vi "AgilentAutoSignalCaptureBinary.vi"() -> ()   [LabVIEW 2016]
uses:
  AgilentControl.ctl
  Channel Config.ctl
  <vilib>/Waveform/WDTOps.llb/WDT Waveform Duration DBL.vi
  <instrlib>/Agilent 6000 Series/Agilent 6000 Series.lvlib
panel:
  out "File Errors":errorcluster
  in  "Shot Notes":string
  out "Last Shot Number":u32
  out "Num Events so far":i32
  out "Last Captured Waveform":waveform(dbl)[](graph)
  in  "Update Graph":bool
  out "Time per acq (ms)":dbl
  out "Elapsed Time (ms)":u32
  in  "Max Waves to capture":i32 min=0 max=1000000 step=1
  in  "Target Data Folder":path=path "C:/test"
  out "Close Error":errorcluster
  in  "stop":bool
  out "Agilent Control Out":T1={"Trig?"=FALSE, "VISA session"="", "Setup to Load"="CH1", "Timeout (ms)"=10000, "Desired Samp"=enum."100", "Captured Samp"=0, "Desired Channels"=[]}
  in  "Agilent Control In":T1={"Trig?"=FALSE, "VISA session"="Agilent6034A", "Setup to Load"="CH1", "Timeout (ms)"=10000, "Desired Samp"=enum."100", "Captured Samp"=2, "Desired Channels"=[]}
  out "Data Download Error":errorcluster[](array[cluster])
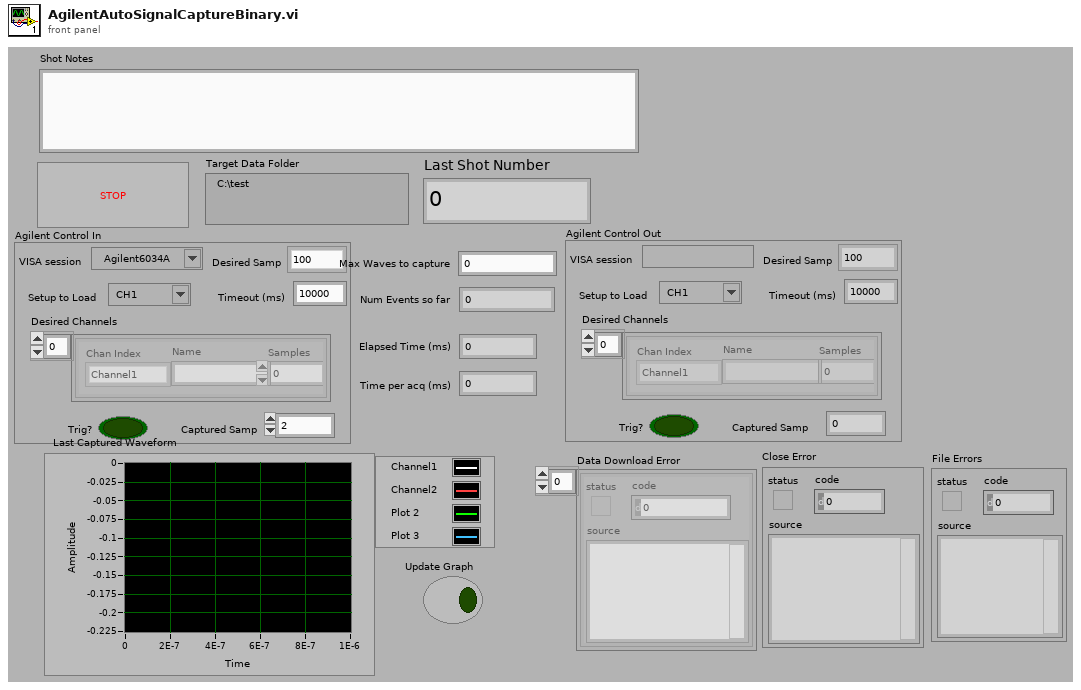
[diagram p1: front panel]
types:
  T1 = typedef "AgilentControl.ctl" = cluster{"Trig?":bool, "VISA session":refnum<visa-resource-name>, "Setup to Load":string, "Timeout (ms)":u32, "Desired Samp":enum32{"100", "250", "500", "1000", "2000", "5000", "10000", "20000", "50000", "100000", "200000", "500000", "1000000", "2000000", "4000000", "8000000"}, "Captured Samp":i32, "Desired Channels":T2[]}
  T2 = typedef "Channel Config.ctl" = cluster{"Chan Index":enum16{"Channel1", "Channel2", "Channel3", "Channel4", "MATH"}, "Name":string, "Samples":i32}
  T3 = enum16{"open", "replace", "create", "open or create", "replace or create", "replace or create with confirmation"}
  T4 = enum32{"100", "250", "500", "1000", "2000", "5000", "10000", "20000", "50000", "100000", "200000", "500000", "1000000", "2000000", "4000000", "8000000"}
  T5 = enum16{"Channel1", "Channel2", "Channel3", "Channel4", "MATH"}
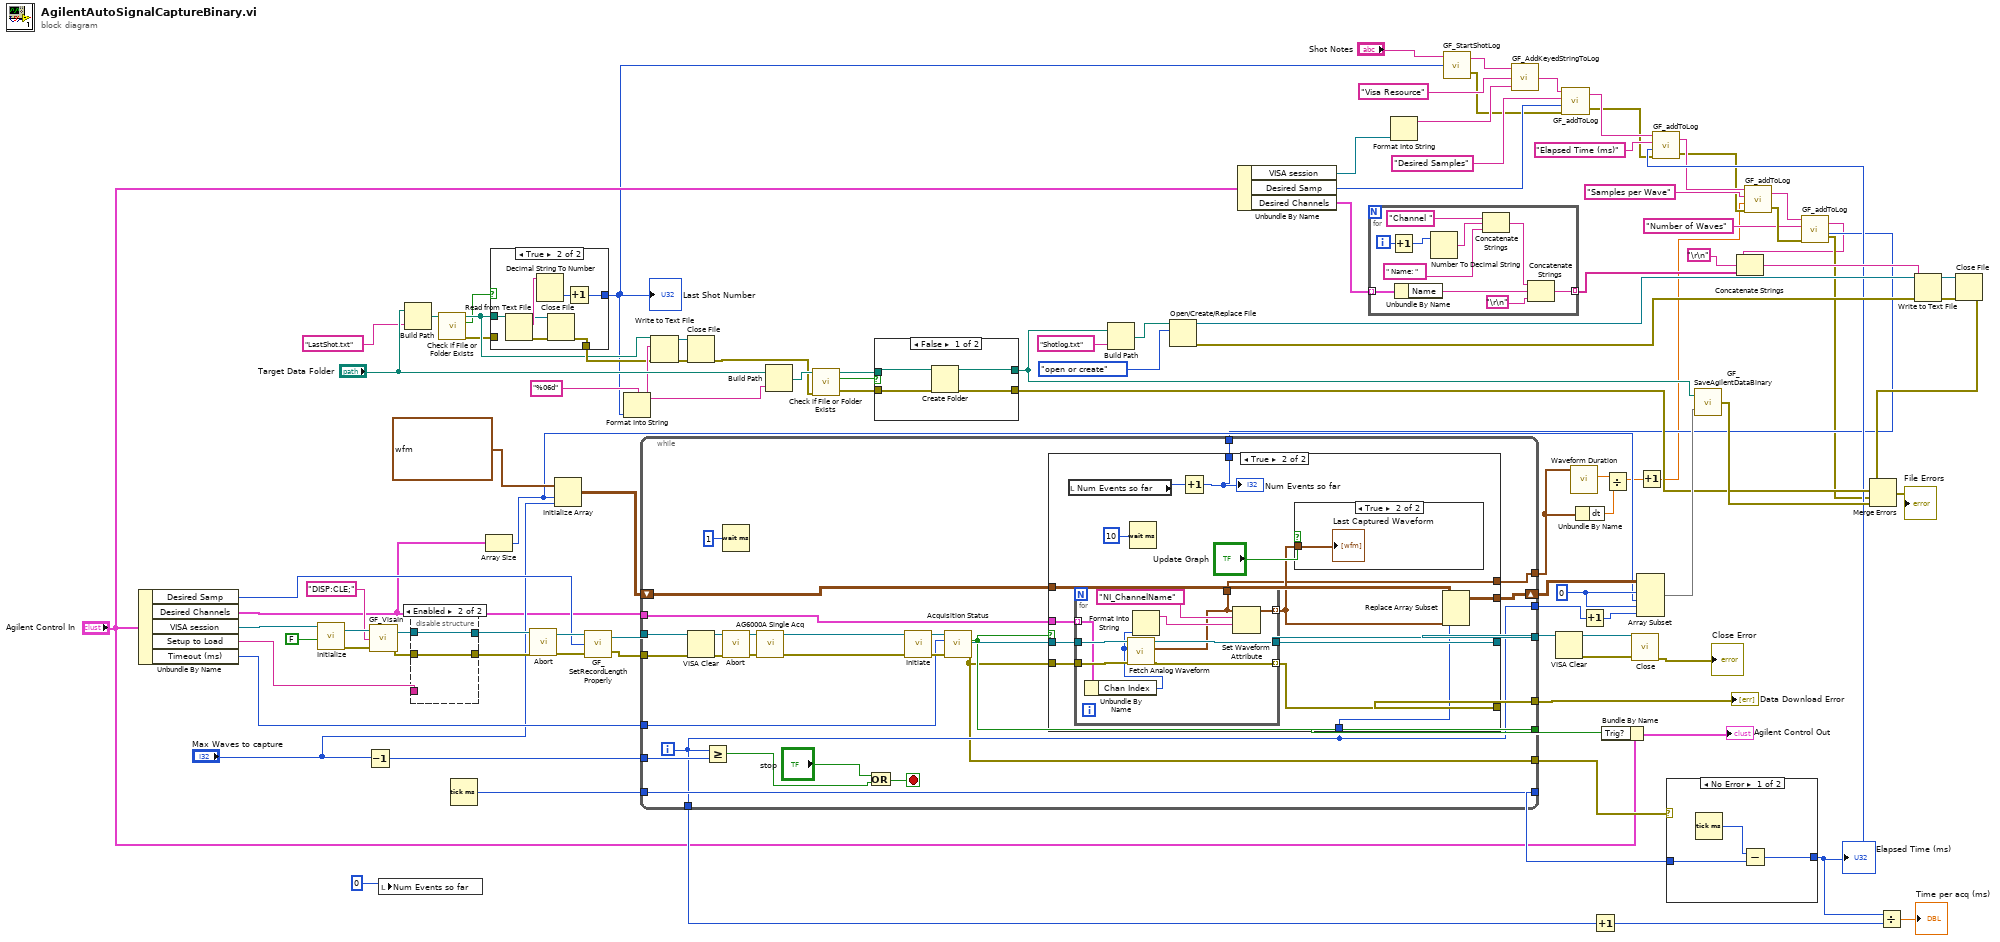
[diagram p0: block diagram]
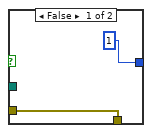
[diagram p2: hidden frame]
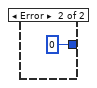
[diagram p4: hidden frame]
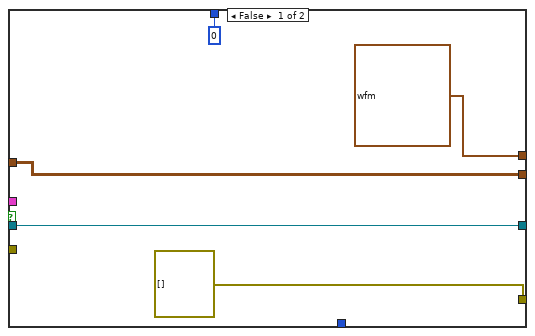
[diagram p5: hidden frame]
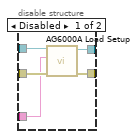
[diagram p7: hidden frame]
diagram:
  w64 = 0 ("index")
  n1 = Unbundle By Name("Agilent Control In") -> ("Desired Samp"=w75:T4, "Desired Channels"=w70:T2[], "VISA session"=w101:refnum<visa-resource-name>, "Setup to Load"=w99:string, "Timeout (ms)"=w98:u32)
  n2 = call <instrlib>:"Initialize.vi"("Reset? (T: Yes)"=FALSE, "VISA resource name"=w101) -> ("error out"=w90:errorcluster, "VISA resource name out"=w91:refnum<visa-resource-name>)  [unwired: 8 in]
  n3 = Decrement(x="Max Waves to capture") -> (x-1=w86:i32)
  n4 = call "GF_VisaIn.vi"("error in (no error)"=w90, "String"="DISP:CLE;", "VISA resource name"=w91) -> ("error out"=w89:errorcluster, "VISA resource name out"=w88:refnum<visa-resource-name>)
  n5 = local write "Num Events so far"(0 ("NumAcq")) -> ()
  n6 = Build Path(base path="Target Data Folder", name or relative path="LastShot.txt") -> (appended path=w33:path)
  n7 = disable-structure shown="Enabled" {
    disable-tunnel: [w107 w108] -> w74
    disable-tunnel: [w106 w109] -> w73
    disable-tunnel: w88 -> [w105 w108]
    disable-tunnel: w89 -> [w104 w109]
    disable-tunnel: w99 -> [w103 _]
    frame Disabled {
      n8 = call "AG6000A Load Setup.vi"("error in (no error)"=w104, "Setup to Load"=w103, "VISA session"=w105) -> ("error out"=w106:errorcluster, "dup VISA session"=w107:refnum<visa-resource-name>)  [unwired: 7 in]
    }
    frame Enabled {
    }
  }
  n9 = call <vilib>:"Check if File or Folder Exists.vi"("path"=w33) -> ("error out"=w30:errorcluster, "file or folder exists?"=w31:bool, "dup path"=w32:path)  [unwired: 8 in]
  n10 = Tick Count (ms)() -> (millisecond timer value=w62:u32)
  n11 = Array Size(array=w70) -> (size(s)=w63:i32)
  n12 = case shown="True" w31 {
    tunnel: [1 w116] -> w28
    tunnel: [w111 w113] -> w34
    tunnel: w32 -> [_ w112]
    tunnel: w30 -> [w111 _]
    frame False {
    }
    frame True {
      n13 = Read from Text File(file (use dialog)=w112) -> (refnum out=w115:refnum<file>, text=w118:string, error out=w114:errorcluster)  [unwired: 3 in, 1 out]
      n14 = Decimal String To Number(string=w118) -> (number=w117:i32)  [unwired: 2 in, 1 out]
      n15 = Close File(refnum=w115, error in=w114) -> (error out=w113:errorcluster)  [unwired: 1 out]
      n16 = Increment(x=w117) -> (x+1=w116:i32)
    }
  }
  "Last Shot Number" <- w28
  n17 = call <instrlib>:"Abort.vi"("error in (no error)"=w73, "VISA resource name"=w74) -> ("error out"=w78:errorcluster, "VISA resource name out"=w79:refnum<visa-resource-name>)  [unwired: 8 in]
  n18 = Initialize Array(waveform(dbl) {"t0"=timestamp(0 s since 1904-01-01), "dt"=1.0, "Y"=[]} ("Waveform Data"), w63, "Max Waves to capture") -> (w72:waveform(dbl)[][])
  n19 = call "GF_SetRecordLengthProperly.vi"("error in (no error)"=w78, "Num Samples"=w75, "VISA resource name"=w79) -> ("error out"=w77:errorcluster, "VISA resource name out"=w76:refnum<visa-resource-name>)
  n20 = Format Into String(format string="%06d", w28) -> (resulting string=w36:string)  [unwired: 2 in, 1 out]
  n21 = while {
    tunnel: [w136] -> w94
    tunnel: [w145] -> w102
    tunnel: w70 -> [w142]
    tunnel: w98 -> [w141]
    tunnel: [w140] -> w97
    tunnel: w76 -> [w135]
    tunnel: w77 -> [w123]
    shift-right: [w125] -> w68
    shift-left: w72 -> [w138]
    tunnel: [w121] -> w85
    tunnel: w86 -> [w130]
    tunnel: w62 -> [w128]
    tunnel: [w128] -> w84
    tunnel: [w124] -> w82
    tunnel: [w124] -> w66
    tunnel: [w120] -> w16
    tunnel: [w119] -> w7
    i -> [w124]
    stop <- w131 stop-if-true
    n22 = VISA Clear(VISA resource name=w135, error in (no error)=w123) -> (VISA resource name out=w134:refnum<visa-resource-name>, error out=w133:errorcluster)
    n23 = Greater Or Equal?(x=w124, y=w130) -> (x >= y?=w129:bool)
    n24 = Wait (ms)(milliseconds to wait=u32 1) -> ()  [unwired: 1 out]
    n25 = call <instrlib>:"Abort.vi"("error in (no error)"=w133, "VISA resource name"=w134) -> ("error out"=w126:errorcluster, "VISA resource name out"=w127:refnum<visa-resource-name>)  [unwired: 8 in]
    n26 = call "AG6000A Single Acq.vi"("error in (no error)"=w126, "VISA session"=w127) -> ("error out"=w122:errorcluster, "dup VISA session"=w139:refnum<visa-resource-name>)  [unwired: 8 in]
    n27 = Or(x="stop", y=w129) -> (x .or. y?=w131:bool)
    n28 = call <instrlib>:"Initiate.vi"("error in (no error)"=w122, "VISA resource name"=w139) -> ("error out"=w143:errorcluster, "VISA resource name out"=w144:refnum<visa-resource-name>)  [unwired: 8 in]
    n29 = call <instrlib>:"Acquisition Status.vi"("error in (no error)"=w143, "Timeout (10000 ms)"=w141, "VISA resource name"=w144) -> ("error out"=w121:errorcluster, "Acquisition Complete?"=w140:bool, "VISA resource name out"=w146:refnum<visa-resource-name>)  [unwired: 6 in]
    n30 = case shown="True" w140 {
      tunnel: w146 -> [w149 w165]
      tunnel: w121 -> [_ w164]
      tunnel: w142 -> [_ w158]
      tunnel: [w149 w163] -> w136
      tunnel: [errorcluster[] [] w162] -> w145
      tunnel: w138 -> [w150 w156]
      tunnel: [w150 w157] -> w125
      tunnel: w124 -> [_ w155]
      tunnel: [waveform(dbl) {"t0"=timestamp(0 s since 1904-01-01), "dt"=1.0, "Y"=[]} ("Waveform Data") w153] -> w120
      tunnel: [0 w152] -> w119
      frame False {
      }
      frame True {
        n31 = local read "Num Events so far"() -> (w159:i32)
        n32 = for {
          tunnel: w165 -> [w176]
          tunnel: w164 -> [w171]
          tunnel: w158 -> [w169] mode=indexing
          tunnel: [w175] -> w163
          tunnel: [w170] -> w162 mode=indexing
          tunnel: [w174] -> w154 mode=indexing
          tunnel: [w167] -> w153
          n33 = Unbundle By Name(w169) -> ("Chan Index"=w168:T5)
          n34 = call <instrlib>:"Fetch Analog Waveform.vi"("error in (no error)"=w171, "Source (0: Channel 1)"=w168, "VISA resource name"=w176) -> ("error out"=w170:errorcluster, "Waveform Data"=w167:waveform(dbl), "VISA resource name out"=w175:refnum<visa-resource-name>)  [unwired: 6 in]
          n35 = Format Into String(w168) -> (resulting string=w172:string)  [unwired: 3 in, 1 out]
          n36 = Set Waveform Attribute(5:w172, 6:"NI_ChannelName" ("name"), 7:w167) -> (3:w174:waveform(dbl))  [unwired: 1 in, 2 out]
        }
        n37 = Wait (ms)(milliseconds to wait=u32 10) -> ()  [unwired: 1 out]
        n38 = Increment(x=w159) -> (x+1=w152:i32)
        "Num Events so far" <- w152
        n39 = case shown="True" "Update Graph" {
          tunnel: w154 -> [_ w166]
          frame False {
          }
          frame True {
            "Last Captured Waveform" <- w166
          }
        }
        n40 = Replace Array Subset(array=w156, new element=w154, index (col)=w155) -> (w157:waveform(dbl)[][])  [unwired: 1 in]
      }
    }
  }
  "Data Download Error" <- w102
  n41 = Write to Text File(file (use dialog)=w32, text=w36, error in=w34) -> (refnum out=w39:refnum<file>, error out=w38:errorcluster)  [unwired: 1 in, 1 out]
  n42 = Close File(refnum=w39, error in=w38) -> (error out=w37:errorcluster)  [unwired: 1 out]
  n43 = Build Path(base path="Target Data Folder", name or relative path=w36) -> (appended path=w60:path)
  n44 = call <vilib>:"Check if File or Folder Exists.vi"("error in (no error)"=w37, "path"=w60) -> ("error out"=w57:errorcluster, "file or folder exists?"=w59:bool, "dup path"=w58:path)  [unwired: 7 in]
  n45 = case shown="False" w59 {
    tunnel: w58 -> [w180 w182]
    tunnel: [w179 w182] -> w56
    tunnel: w57 -> [w178 w181]
    tunnel: [w177 w181] -> w53
    frame False {
      n46 = Create Folder(path (use dialog)=w180, error in=w178) -> (created path=w179:path, error out=w177:errorcluster)  [unwired: 1 in, 1 out]
    }
    frame True {
    }
  }
  n47 = Build Path(base path=w56, name or relative path="Shotlog.txt") -> (appended path=w50:path)
  n48 = Open/Create/Replace File(file path (use dialog)=w50, operation (0:open)=T3."open or create") -> (refnum out=w48:refnum<file>, error out=w35:errorcluster)  [unwired: 4 in, 1 out]
  n49 = Unbundle By Name("Agilent Control In") -> ("VISA session"=w42:refnum<visa-resource-name>, "Desired Samp"=w22:T4, "Desired Channels"=w43:T2[])
  n50 = for {
    tunnel: w43 -> [w185] mode=indexing
    tunnel: [w189] -> w4 mode=indexing
    i -> [w187]
    n51 = Increment(x=w187) -> (x+1=w186:i32)
    n52 = Unbundle By Name(w185) -> ("Name"=w183:string)
    n53 = Number To Decimal String(number=w186) -> (decimal integer string=w191:string)  [unwired: 1 in]
    n54 = Concatenate Strings("Channel " ("initial string"), w191, " Name: " ("string")) -> (w184:string)
    n55 = Concatenate Strings(w184, w183, "\r\n") -> (w189:string)
  }
  n56 = Format Into String(w42) -> (resulting string=w25:string)  [unwired: 3 in, 1 out]
  n57 = call "GF_StartShotLog.vi"("Shot Number"=w28, "Shot Notes"="Shot Notes") -> ("error out"=w11:errorcluster, "Shotlog Beginning"=w27:string)  [unwired: 1 in]
  n58 = call "GF_AddKeyedStringToLog.vi"("Value String"=w25, "Key Name"="Visa Resource" ("string"), "Current Log"=w27) -> ("concatenated string"=w24:string)
  n59 = VISA Clear(VISA resource name=w94) -> (VISA resource name out=w93:refnum<visa-resource-name>, error out=w92:errorcluster)  [unwired: 1 in]
  n60 = call "GF_addToLog.vi"("error in"=w11, "Value"=w22, "Key Name"="Desired Samples" ("string"), "Current String"=w24) -> ("error out"=w12:errorcluster, "concatenated string"=w21:string)
  n61 = call-poly <vilib>:"Waveform Duration.vi"("waveform in"=w16) -> ("duration"=w15:dbl)  [unwired: 8 in, 2 out]
  n62 = Unbundle By Name(w16) -> ("dt"=w14:dbl)
  n63 = Increment(x=w66) -> (x+1=w65:i32)
  n64 = Increment(x=w82) -> (x+1=w83:i32)
  n65 = Bundle By Name(cluster="Agilent Control In", "Trig?"=w97) -> (→"Agilent Control Out":T1)
  n66 = Divide(x=w15, y=w14) -> (x/y=w2:dbl)
  n67 = call <instrlib>:"Close.vi"("error in (no error)"=w92, "VISA resource name"=w93) -> ("error out"=→"Close Error":errorcluster)  [unwired: 9 in]
  n68 = Array Subset(array=w68, index (row)=w64, length (row)=w63, index (col)=w64, length (col)=w65) -> (w67:waveform(dbl)[][])
  n69 = Increment(x=w2) -> (x+1=w1:dbl)
  n70 = case shown="No Error" w85 {
    tunnel: w84 -> [w194 _]
    tunnel: [w193 u32 0] -> w19
    frame No Error {
      n71 = Tick Count (ms)() -> (millisecond timer value=w195:u32)
      n72 = Subtract(x=w195, y=w194) -> (x-y=w193:u32)
    }
    frame Error {
    }
  }
  "Elapsed Time (ms)" <- w19
  n73 = call "GF_addToLog.vi"("error in"=w12, "Value"=w19, "Key Name"="Elapsed Time (ms)", "Current String"=w21) -> ("error out"=w13:errorcluster, "concatenated string"=w18:string)
  n74 = call "GF_SaveAgilentDataBinary.vi"("Array"=w67, "Base Path"=w56) -> ("File Write Errors"=w54:errorcluster[])
  n75 = call "GF_addToLog.vi"("error in"=w13, "Value"=w1, "Key Name"="Samples per Wave", "Current String"=w18) -> ("error out"=w9:errorcluster, "concatenated string"=w10:string)
  n76 = call "GF_addToLog.vi"("error in"=w9, "Value"=w7, "Key Name"="Number of Waves", "Current String"=w10) -> ("error out"=w6:errorcluster, "concatenated string"=w5:string)
  n77 = Concatenate Strings(w5, "\r\n", w4) -> (w51:string)
  n78 = Divide(x=w19, y=w83) -> (x/y=→"Time per acq (ms)":dbl)
  n79 = Write to Text File(file (use dialog)=w48, text=w51, error in=w35) -> (refnum out=w47:refnum<file>, error out=w46:errorcluster)  [unwired: 1 in, 1 out]
  n80 = Close File(refnum=w47, error in=w46) -> (error out=w45:errorcluster)  [unwired: 1 out]
  n81 = Merge Errors(w45, w53, w6, w54) -> (→"File Errors":errorcluster)
